vi "SetNag_Commands.vi"() -> ()   [LabVIEW 2013]
panel:
  out "unsigned byte array":u8[](array[numeric])
  out "error code":i32
  out "byte count":u32
  in  "Go":bool
  out "Read":string
  in  "Write":string
  in  "Quit":bool
  in  "Com Port":i32(ring) items=["Com 1", "Com 2", "Com 3", "Com 4", "Com 5", "Com 6", "COM 7", "COM 8", "COM 9", "COM 10", "COM 11", "COM 12", "com 13", "COM 14"]
  in  "Baud Rate":i32(ring)=2 items=["2400", "4800", "9600", "19200", "38400", "57600", "115200"]
  # "Instructions:\nEnter SetNag command as outlined in SetNag manual\non page 41. Begin command with \"_\" and end with \"\\r\".\nFor example, command _OXY will be written as \"_OXY\\r\". \nWrite command then press GO."
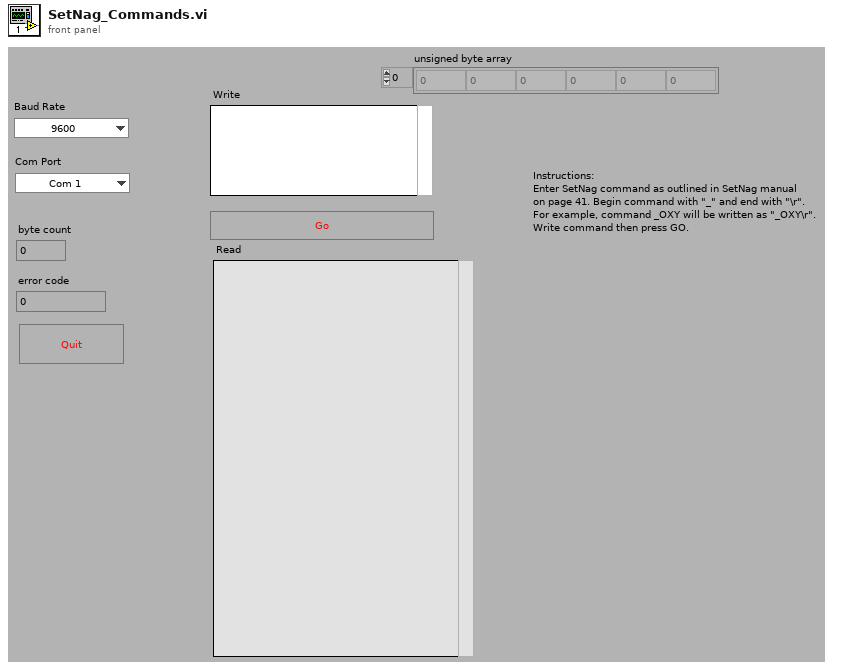
[diagram p1: front panel]
types:
  T1 = enum16{"no parity", "odd parity", "even parity", "mark parity", "space parity"}
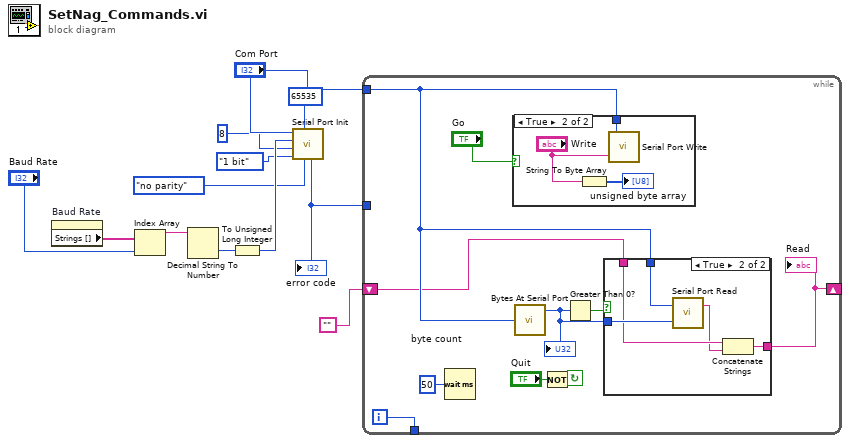
[diagram p0: block diagram]
diagram:
  n1 = property on="Baud Rate" class="Ring (strict)"() -> ("Strings []"=w9:string[])  [unwired: 2 in, 2 out]
  n2 = Index Array(array=w9, index="Baud Rate") -> (element=w8:string)
  n3 = Decimal String To Number(string=w8) -> (number=w10:i32)  [unwired: 2 in, 1 out]
  n4 = To Unsigned Long Integer(number=w10) -> (unsigned 32bit integer=w7:u32)
  n5 = call <vilib>:"Serial Port Init.vi"("parity"=T1."no parity", "buffer size"=u16 65535, "stop bits"=enum16{"1 bit", "1.5 bits", "2 bits"}."1 bit", "data bits"=u16 8, "baud rate"=w7, "port number"="Com Port") -> ("error code"=w5:i32)  [unwired: 1 in]
  "error code" <- w5
  n6 = while {
    tunnel: [w14] -> _
    shift-left: "" -> [w15]
    shift-right: [w13] -> _
    tunnel: w5 -> [_]
    tunnel: "Com Port" -> [w19]
    i -> [w14]
    stop <- w16 continue-if-true
    n7 = Wait (ms)(milliseconds to wait=u32 50) -> ()  [unwired: 1 out]
    n8 = case shown="True" "Go" {
      tunnel: w19 -> [_ w31]
      frame False {
      }
      frame True {
        n9 = String To Byte Array(string="Write") -> (unsigned byte array=→"unsigned byte array":u8[])
        n10 = call <vilib>:"Serial Port Write.vi"("string to write"="Write", "port number"=w31) -> ()  [unwired: 1 out]
      }
    }
    n11 = call <vilib>:"Bytes At Serial Port.vi"("port number"=w19) -> ("byte count"=w18:u32)  [unwired: 1 out]
    "byte count" <- w18
    n12 = Not(x="Quit") -> (.not. x?=w16:bool)
    n13 = Greater Than 0?(x=w18) -> (x > 0?=w20:bool)
    n14 = case shown="True" w20 {
      tunnel: w19 -> [_ w28]
      tunnel: w18 -> [_ w27]
      tunnel: w15 -> [w23 w26]
      tunnel: [w23 w24] -> w13
      frame False {
      }
      frame True {
        n15 = call <vilib>:"Serial Port Read.vi"("requested byte count"=w27, "port number"=w28) -> ("string read"=w25:string)  [unwired: 1 out]
        n16 = Concatenate Strings(w26, w25) -> (w24:string)
      }
    }
    "Read" <- w13
  }
